vi "SenderTCP.vi"() -> ()   [LabVIEW 2023]
uses:
  <vilib>/numeric/sub_Random U32.vi
  <vilib>/numeric/Random Number (Range) U64.vi
panel:
  out "bytes written":i32
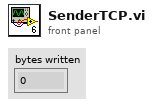
[diagram p1: front panel]
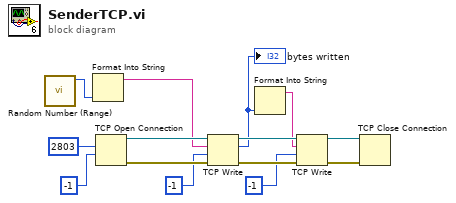
[diagram p0: block diagram]
diagram:
  n1 = call-poly <vilib>:"Random Number (Range).vi"() -> ("number"=w11:u64)  [unwired: 11 in]
  n2 = Format Into String(w11) -> (resulting string=w10:string)  [unwired: 3 in, 1 out]
  n3 = TCP Open Connection(remote port or service name=u16 2803 ("port"), timeout ms (60000)=-1) -> (connection ID=w13:refnum<k5>, error out=w12:errorcluster)  [unwired: 3 in]
  n4 = TCP Write(connection ID=w13, data in=w10, error in (no error)=w12, 9:-1 ("timeout ms (25000)")) -> (connection ID out=w7:refnum<k5>, bytes written=w1:i32, error out=w6:errorcluster)
  "bytes written" <- w1
  n5 = Format Into String(w1) -> (resulting string=w3:string)  [unwired: 3 in, 1 out]
  n6 = TCP Write(connection ID=w7, data in=w3, error in (no error)=w6, 9:-1 ("timeout ms (25000)")) -> (connection ID out=w4:refnum<k5>, error out=w5:errorcluster)  [unwired: 1 out]
  n7 = TCP Close Connection(connection ID=w4, error in (no error)=w5) -> ()  [unwired: 1 in, 2 out]
